vi "FRCts20_EspEngine_InitSearchBrowser.vi"(8 "error in (no error)":errorcluster, 9 "select-choice-location":string, 10 "select-choice-software":string, 11 "httpRequestID":u32) -> (0 "error out":errorcluster, 2 "SearchBrowser":T2, 3 "httpRequestID out":u32)   [LabVIEW 2014, in "FRCts20_EspEngine.lvlib"]
uses:
  FRCts20_EspEngine.lvlib
  TypeDefs/FRCts20_EspEngine_SearchBrowser.ctl
  Backend/source/VI Source/FRCts20_Backend_API/FRCts20_Backend_API_EventRoot.ctl
  Backend/source/VI Source/FRCts20_Backend_API/FRCts20_Backend_API_Command_EventRoot.ctl
  Backend/source/VI Source/FRCts20_Backend_API/FRCts20_Backend_API_EventRoot.vi
  Backend/source/VI Source/FRCts20_Backend_API/FRCts20_Backend_API.lvlib
  Web Methods/source/VI Source/FRCts20_WebMethods.lvlib
panel:
  in  "EventRoot Out":T1
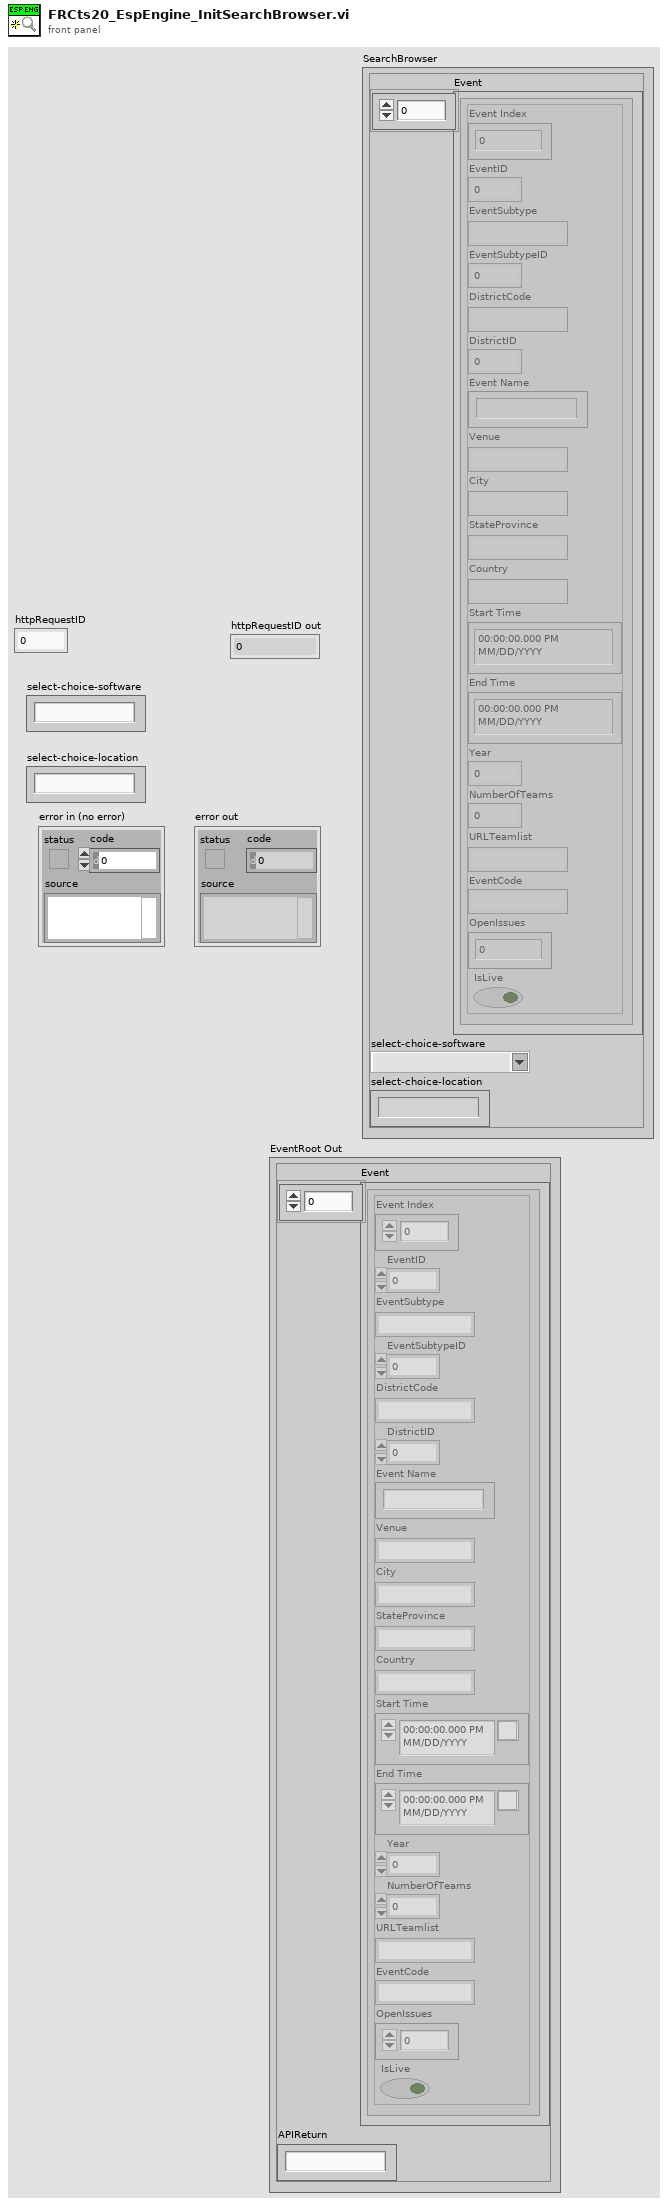
[diagram p1: front panel]
types:
  T1 = typedef "FRCts20_Backend_API.lvlib/FRCts20_Backend_API_EventRoot.ctl" = cluster{"Event":cluster{"Event Index":u32, "EventID":u32, "EventSubtype":string, "EventSubtypeID":u32, "DistrictCode":string, "DistrictID":u32, "Event Name":string, "Venue":string, "City":string, "StateProvince":string, "Country":string, "Start Time":timestamp, "End Time":timestamp, "Year":u32, "NumberOfTeams":u32, "URLTeamlist":string, "EventCode":string, "OpenIssues":u8, "IsLive":bool}[], "APIReturn":string}
  T2 = typedef "FRCts20_EspEngine.lvlib/FRCts20_EspEngine_SearchBrowser.ctl" = cluster{"Event":cluster{"Event Index":u32, "EventID":u32, "EventSubtype":string, "EventSubtypeID":u32, "DistrictCode":string, "DistrictID":u32, "Event Name":string, "Venue":string, "City":string, "StateProvince":string, "Country":string, "Start Time":timestamp, "End Time":timestamp, "Year":u32, "NumberOfTeams":u32, "URLTeamlist":string, "EventCode":string, "OpenIssues":u8, "IsLive":bool}[], "select-choice-software":string, "select-choice-location":string}
  T3 = typedef "FRCts20_Backend_API.lvlib/FRCts20_Backend_API_Command_EventRoot.ctl" = string
  T4 = cluster{"Event Index":u32, "EventID":u32, "EventSubtype":string, "EventSubtypeID":u32, "DistrictCode":string, "DistrictID":u32, "Event Name":string, "Venue":string, "City":string, "StateProvince":string, "Country":string, "Start Time":timestamp, "End Time":timestamp, "Year":u32, "NumberOfTeams":u32, "URLTeamlist":string, "EventCode":string, "OpenIssues":u8, "IsLive":bool}[]
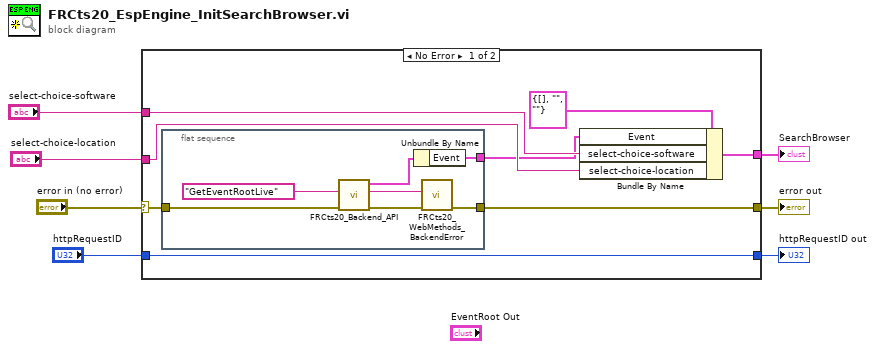
[diagram p0: block diagram]
diagram:
  n1 = case shown="No Error" "error in (no error)" {
    selector: "error in (no error)" -> [w11 w23]
    tunnel: [w10 w23] -> w7
    tunnel: [w13 _] -> w5
    tunnel: "httpRequestID" -> [w12 _]
    tunnel: "select-choice-software" -> [w15 _]
    tunnel: "select-choice-location" -> [w14 _]
    tunnel: [w12 _] -> w1
    frame No Error {
      n2 = flat-sequence {
        tunnel: w11 -> [w20]
        tunnel: [w19] -> w10
        tunnel: [w16] -> w9
        frame #0 {
          n3 = call-poly "FRCts20_Backend_API.vi"("error in (no error)"=w20, "Message"=T3 "GetEventRootLive") -> ("error out"=w22:errorcluster, "Status"=w21:string, "EventRoot Out"=w18:T1)  [unwired: 7 in]
          n4 = Unbundle By Name(w18) -> ("Event"=w16:T4)
          n5 = call "FRCts20_WebMethods_BackendError.vi"("error in (no error)"=w22, "Status"=w21) -> ("error out"=w19:errorcluster)  [unwired: 8 in, 1 out]
        }
      }
      n6 = Bundle By Name(cluster=T2 {"Event"=[], "select-choice-software"="", "select-choice-location"=""} ("SearchBrowser"), "Event"=w9, "select-choice-software"=w15, "select-choice-location"=w14) -> (w13:T2)
    }
    frame Error {
    }
  }
  "error out" <- w7
  "SearchBrowser" <- w5
  "httpRequestID out" <- w1
